vi "Decompose VI (Refnum).vi"(8 "Error in":errorcluster caption="Error in (no error)", 11 "VI Refnum":refnum<vi>) -> (0 "Error out":errorcluster, 1 "Block Diagram XML":string, 2 "Front Panel XML":string, 3 "VI Refnum Out":refnum<vi>, 4 "Other resources":T1)   [LabVIEW 2018, in "Resource Manipulation.lvlib"]
uses:
  Resource Manipulation.lvlib
  Resource Array.ctl
  Resource.ctl
  <vilib>/Utility/error.llb/Error Cluster From Error Code.vi
  Find Resource by Type (String).vi
  <vilib>/ErrorRing/Error Ring.xnode
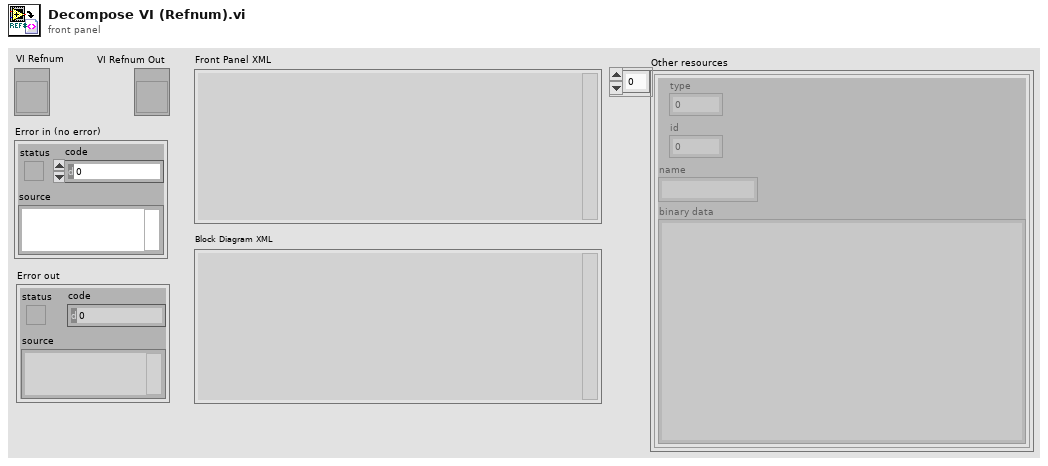
[diagram p1: front panel]
types:
  T1 = typedef "Resource Manipulation.lvlib/Resource Array.ctl" = T2[]
  T2 = typedef "Resource Manipulation.lvlib/Resource.ctl" = cluster{"type":u32, "id":i32, "name":string, "binary data":string}
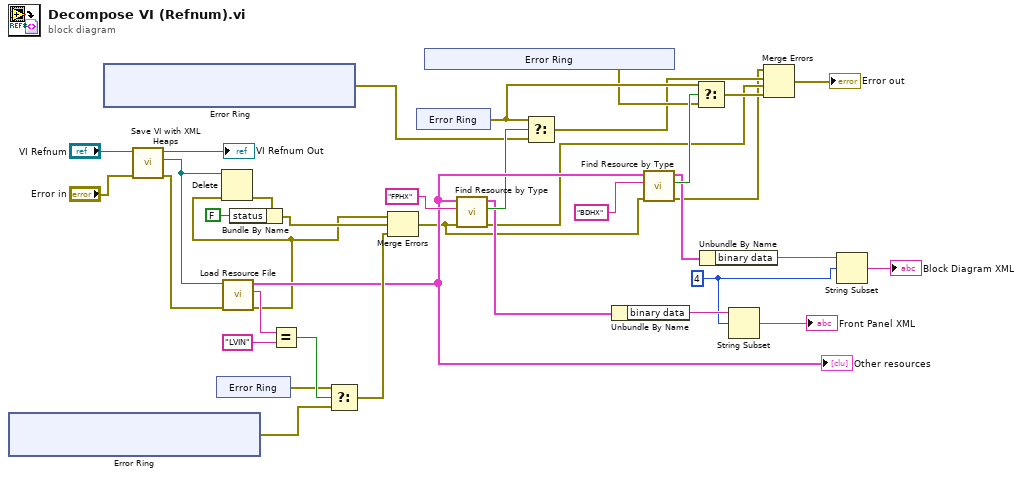
[diagram p0: block diagram]
diagram:
  w4 = 4
  n1 = xnode "Error Ring"() -> ("error out"=w25:errorcluster)
  n2 = xnode "Error Ring"() -> ("error out"=w20:errorcluster)
  n3 = call "Save VI with XML Heaps.vi"("error in (no error)"="Error in", "VI Refnum In"="VI Refnum") -> ("error out"=w33:errorcluster, "VI Path out"=w32:path, "VI Refnum Out"=→"VI Refnum Out":refnum<vi>)  [unwired: 7 in]
  n4 = xnode "Error Ring"() -> ("error out"=w26:errorcluster)
  n5 = call "Load Resource File.vi"("error in (no error)"=w33, "Resource file"=w32) -> ("error out"=w2:errorcluster, "File Type"=w29:string, "Resources"=w22:T1)  [unwired: 7 in]
  "Other resources" <- w22
  n6 = Delete(path (use dialog)=w32, error in=w2) -> (error out=w31:errorcluster)  [unwired: 3 in, 2 out]
  n7 = Bundle By Name(cluster=w31, "status"=FALSE) -> (w3:errorcluster)
  n8 = Equal?(x=w29, y="LVIN") -> (x = y?=w27:bool)
  n9 = Select(t=w26, s=w27, f=w25) -> (s? t:f=w24:errorcluster)
  n10 = Merge Errors(w2, w3, w24) -> (w8:errorcluster)
  n11 = xnode "Error Ring"() -> ("error out"=w18:errorcluster)
  n12 = xnode "Error Ring"() -> ("error out"=w17:errorcluster)
  n13 = call-poly "Find Resource by Type.vi"("Error in"=w8, "Resource Type"="FPHX", "Resources"=w22) -> ("Error out"=w5:errorcluster, "Found?"=w21:bool, "Resource"=w15:T2)  [unwired: 5 in, 1 out]
  n14 = Select(t=w18, s=w21, f=w20) -> (s? t:f=w6:errorcluster)
  n15 = Unbundle By Name(w15) -> ("binary data"=w13:string)
  n16 = call-poly "Find Resource by Type.vi"("Error in"=w8, "Resource Type"="BDHX", "Resources"=w22) -> ("Error out"=w1:errorcluster, "Found?"=w19:bool, "Resource"=w14:T2)  [unwired: 5 in, 1 out]
  n17 = Select(t=w18, s=w19, f=w17) -> (s? t:f=w7:errorcluster)
  n18 = Unbundle By Name(w14) -> ("binary data"=w12:string)
  n19 = String Subset(string=w13, offset (0)=w4) -> (substring=→"Front Panel XML":string)  [unwired: 1 in]
  n20 = Merge Errors(w1, w6, w5, w7) -> (→"Error out":errorcluster)
  n21 = String Subset(string=w12, offset (0)=w4) -> (substring=→"Block Diagram XML":string)  [unwired: 1 in]
